vi "New Missing VI.vi"(8 "error in (no error)":errorcluster, 10 "App Refnum":refnum<vi>, 11 "SubVI Refnum":refnum<vi>) -> (0 "error out":errorcluster, 3 "Missing VI Type out":refnum<class "Missing VI Type.lvclass">)   [LabVIEW 2020, in "Peek Window.lvlib" / "Missing VI Type.lvclass"]
uses:
  Missing VI Type.lvclass
  D:/Code/VI-Peek/source/Peek Window/VI Types/Standard VI Type/Standard VI Type.lvclass
  Standard VI Type/Standard VI Type.lvclass/Standard VI Type.ctl
  Standard VI Type/Write App Refnum.vi
  Standard VI Type/Write Full Qualified Name.vi
  Standard VI Type/Write Openable.vi
  Standard VI Type/Write Selectable.vi
  Missing VI Type.lvclass/Missing VI Type.ctl
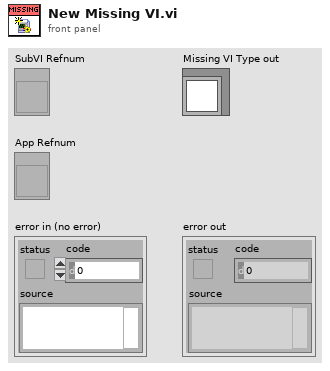
[diagram p1: front panel]
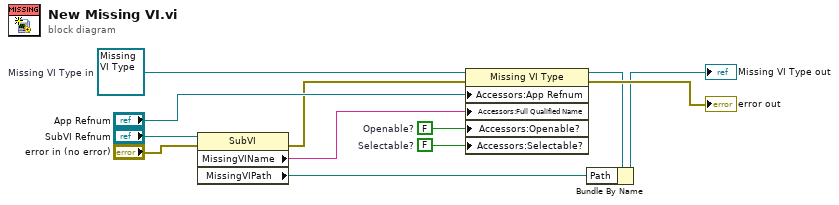
[diagram p0: block diagram]
diagram:
  w4 = FALSE  # Selectable?
  w5 = FALSE  # Openable?
  w12 = refnum<class "Missing VI Type.lvclass"> refnum  # Missing VI Type in
  n1 = property class="SubVI"(reference="SubVI Refnum", error in="error in (no error)") -> (error out=w6:errorcluster, "MissingVIName"=w8:string, "MissingVIPath"=w1:path)  [unwired: 1 out]
  n2 = property class="Missing VI Type"(reference=w12, error in=w6, "Accessors:App Refnum"="App Refnum", "Accessors:Full Qualified Name"=w8, "Accessors:Openable?"=w5, "Accessors:Selectable?"=w4) -> (reference out=w3:refnum<class "Missing VI Type.lvclass">, error out=→"error out":errorcluster)
  n3 = Bundle By Name(cluster=w3, "Path"=w1) -> (→"Missing VI Type out":refnum<class "Missing VI Type.lvclass">)
